vi "DefaultUserSettings Full Path.vi"() -> (3 "DefaultUserSettings Full Path":path)   [LabVIEW 2020, in "User Preferences File.lvclass"]
doc: "Location of the DefaultUserSettings.ini configuration file."
uses:
  User Preferences File.lvclass
  File IO/Project Locations/Project Locations.lvlib
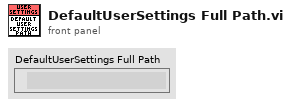
[diagram p1: front panel]
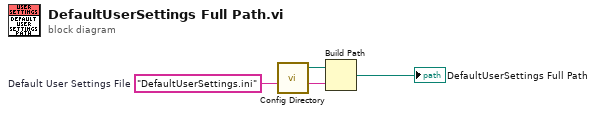
[diagram p0: block diagram]
diagram:
  w3 = "DefaultUserSettings.ini"  # Default User Settings File
  n1 = call "Config Directory.vi"() -> ("Config Directory"=w2:path)  [unwired: 2 in]
  n2 = Build Path(base path=w2, name or relative path=w3) -> (appended path=→"DefaultUserSettings Full Path":path)
